vi "create timestamp text file (seconds for HHMMSS.SSS)(SubVI).vi"(8 "error in":errorcluster, 9 "time offset":dbl, 10 "Array":dbl[](array[numeric]), 11 "appended path":path) -> (0 "error out":errorcluster)   [LabVIEW 2024]
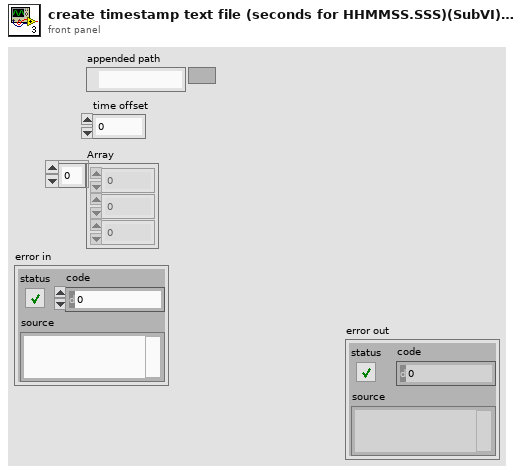
[diagram p1: front panel]
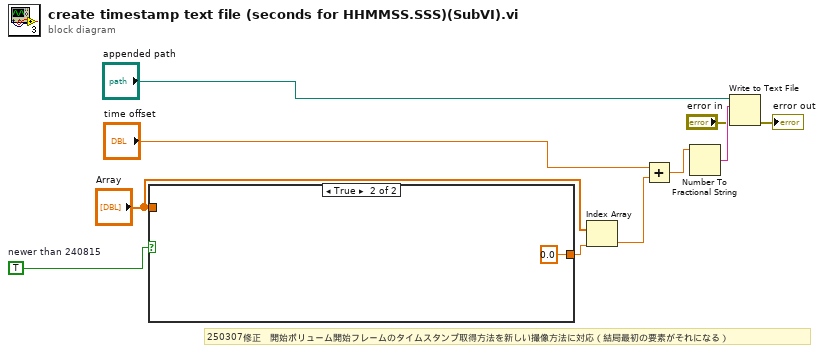
[diagram p0: block diagram]
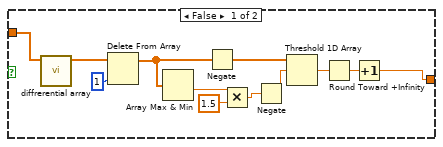
[diagram p2: hidden frame]
diagram:
  w3 = TRUE  # newer than 240815
  # "250307修正　開始ボリューム開始フレームのタイムスタンプ取得方法を新しい撮像方法に対応（結局最初の要素がそれになる）"
  n1 = case shown="True" w3 {
    tunnel: "Array" -> [w12 _]
    tunnel: [w11 0.0] -> w2
    frame False {
      n2 = call "diffrerential array.vi"("Array in"=w12) -> ("Array"=w13:dbl[])  [unwired: 10 in]
      n3 = Delete From Array(array=w13, index=1) -> (array with subset deleted=w14:dbl[])  [unwired: 1 in, 1 out]
      n4 = Array Max & Min(array=w14) -> (min value=w21:dbl)  [unwired: 3 out]
      n5 = Negate(x=w14) -> (-x=w16:dbl[])
      n6 = Multiply(x=w21, y=1.5) -> (x*y=w19:dbl)
      n7 = Negate(x=w19) -> (-x=w15:dbl)
      n8 = Threshold 1D Array(2:w15, 3:w16) -> (0:w18:dbl)  [unwired: 1 in]
      n9 = Round Toward +Infinity(x=w18) -> (ceil(x): smallest int >= x=w17:dbl)
      n10 = Increment(x=w17) -> (x+1=w11:dbl)
    }
    frame True {
    }
  }
  n11 = Index Array(array="Array", index=w2) -> (element=w1:dbl)
  n12 = Add(x="time offset", y=w1) -> (x+y=w7:dbl)
  n13 = Number To Fractional String(number=w7) -> (F-format string=w10:string)  [unwired: 3 in]
  n14 = Write to Text File(file (use dialog)="appended path", text=w10, error in="error in") -> (error out=→"error out":errorcluster)  [unwired: 1 in, 2 out]
